vi "GT_GetDi.vi"(4 "diType in":i16(ring) items=["Limit_Positive", "Limit_Negative", "Alarm", "Home", "Gpi", "arrive"], 5 "rtn_In":cluster{"rtn":i16, "Func":string}) -> (0 "IOOut":bool[](array[boolean]), 1 "diType out":i16, 2 "rtn_Out":cluster{"rtn":i16, "Func":string})   [LabVIEW 2014]
uses:
  VC6/gts.dll
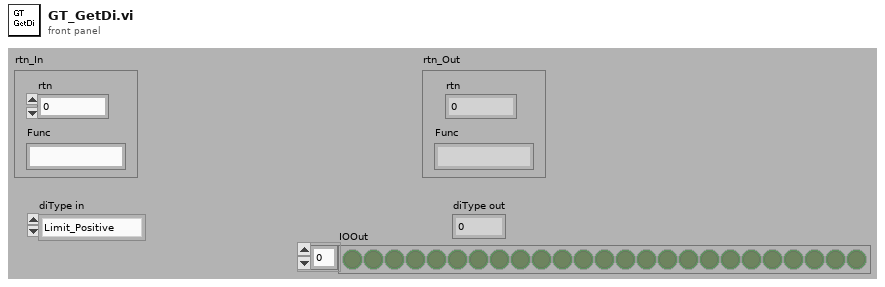
[diagram p1: front panel]
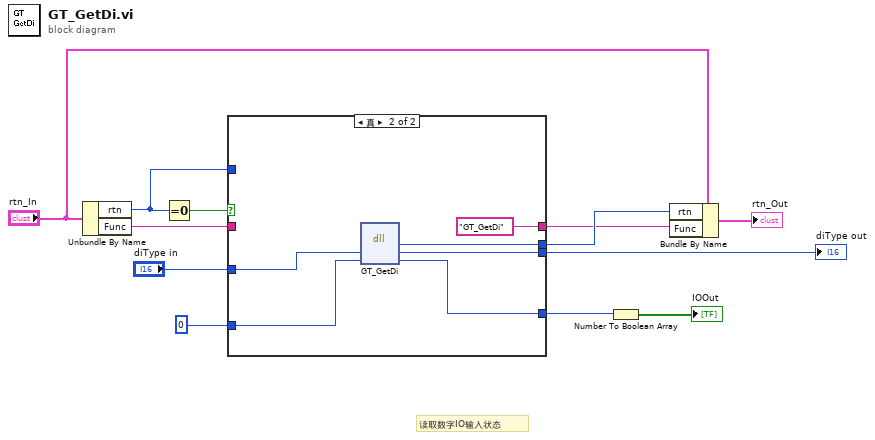
[diagram p0: block diagram]
diagram:
  # "读取数字IO输入状态"
  n1 = Unbundle By Name("rtn_In") -> ("rtn"=w5:i16, "Func"=w6:string)
  n2 = Equal To 0?(x=w5) -> (x = 0?=w12:bool)
  n3 = case shown="真" w12 {
    tunnel: "diType in" -> [w14 w22]
    tunnel: 0 ("pValue") -> [w13 w21]
    tunnel: [w15 w20] -> w8
    tunnel: [w16 "GT_GetDi" ("Func")] -> w7
    tunnel: w6 -> [w16 _]
    tunnel: w5 -> [w15 _]
    tunnel: [w14 w18] -> w4
    tunnel: [w13 w17] -> w3
    frame False {
    }
    frame True {
      n4 = dll-call lib="PTH2Fabs DNewGTS AC-800LWin7版源程序-20170926gts85VC6gts.dll" fn="GT_GetDi"("diType"=w22, "pValue"=w21) -> ("rtn"=w20:i16, "diType"=w18:i16, "pValue"=w17:i32)  [unwired: 3 in, 2 out]
    }
  }
  "diType out" <- w4
  n5 = Number To Boolean Array(number=w3) -> (Boolean array=→"IOOut":bool[])
  n6 = Bundle By Name(cluster="rtn_In", "rtn"=w8, "Func"=w7) -> (→"rtn_Out":cluster{"rtn":i16, "Func":string})
